vi "ActionVIOnCompile.vi"(8 "error in (no error)":errorcluster, 11 "Device Item Ref in":T1 format="%.0x") -> (0 "error out":errorcluster)   [LabVIEW 2020, in "PXI-2514 System Explorer.lvlib"]
uses:
  PXI-2514 System Explorer.lvlib
  <vilib>/NI VeriStand/Custom Device API/Custom Device Item Ref.ctl
  Shared/Compiled.Settings.ctl
  Shared/Constants.vi
  <vilib>/NI VeriStand/Custom Device API/Get Item Property (U16).vi
  <vilib>/NI VeriStand/Custom Device API/Get Item Property (String).vi
  <vilib>/NI VeriStand/Custom Device Tools/Custom Device Utility Library/NI VeriStand - Search for Item by Name.vi
  <vilib>/NI VeriStand/Custom Device API/Set Item Property (Variant).vi
  <vilib>/NI VeriStand/Custom Device Tools/Custom Device Utility Library/Custom Device Utility Library.lvlib
  <vilib>/NI VeriStand/Custom Device API/Custom Device API.lvlib
  <vilib>/NI/NIVS Inline Async API/_Data Access System Explorer/Data Access System Explorer.lvlib
  Shared/PXI-2514 Shared.lvlib
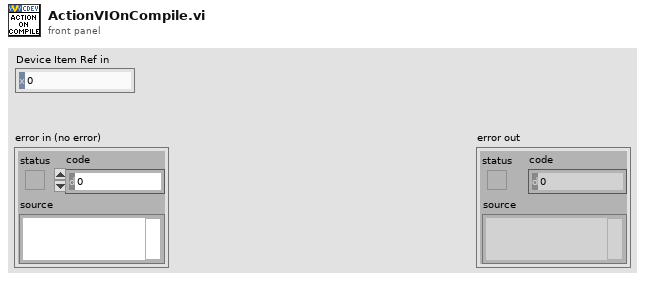
[diagram p1: front panel]
types:
  T1 = typedef "Custom Device API.lvlib/Custom Device Item Ref.ctl" = u64
  T2 = cluster{"Name":string, "Type":enum16{"Output/Write", "Input/Read", "Input/ReadWrite"}, "VS Refs":T1[]}
  T3 = enum16{"Output/Write", "Input/Read", "Input/ReadWrite"}
  T4 = typedef "PXI-2514 Shared.lvlib/Compiled.Settings.ctl" = cluster{"Name":string, "Async Init Timeout":u16, "Hardware Device Name":string}
  T5 = typedef "Custom Device API.lvlib/Custom Device Item Info.ctl" = cluster{"Name":string, "Is Channel":bool, "GUID":string, "Is Waveform":bool}
  T6 = cluster{"Name":string, "Type":enum16{"Output/Write", "Input/Read", "Input/ReadWrite"}, "VS Refs":T1[]}[]
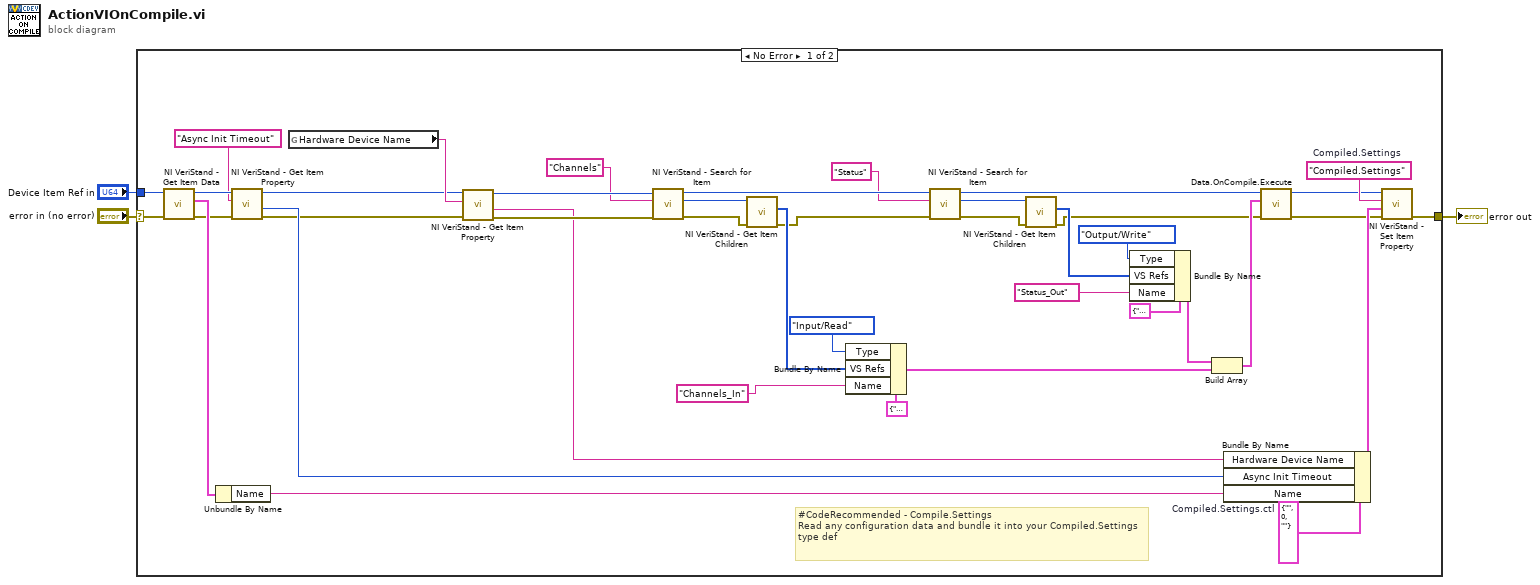
[diagram p0: block diagram]
diagram:
  n1 = case shown="No Error" "error in (no error)" {
    selector: "error in (no error)" -> [w37 w45]
    tunnel: [w38 w45] -> w2
    tunnel: "Device Item Ref in" -> [w36 _]
    frame No Error {
      w17 = T4 {"Name"="", "Async Init Timeout"=0, "Hardware Device Name"=""}  # Compiled.Settings.ctl
      w40 = "Compiled.Settings"  # Compiled.Settings
      # "#CodeRecommended - Compile.Settings\nRead any configuration data and bundle it into your Compiled.Settings type def"
      n2 = call <vilib>:"NI VeriStand - Get Item Data.vi"("error in (no error)"=w37, "Item Ref in"=w36) -> ("error out"=w16:errorcluster, "Item Info"=w35:T5, "Item Ref out"=w15:T1)  [unwired: 6 in, 1 out]
      n3 = Unbundle By Name(w35) -> ("Name"=w34:string)
      n4 = call-poly <vilib>:"NI VeriStand - Get Item Property.vi"("error in (no error)"=w16, "Property Name"="Async Init Timeout", "Item Ref in"=w15) -> ("error out"=w9:errorcluster, "Value"=w13:u16, "Item Ref out"=w11:T1)  [unwired: 5 in, 1 out]
      n5 = global read "Constants.vi" "Hardware Device Name"() -> (w12:string)
      n6 = call-poly <vilib>:"NI VeriStand - Get Item Property.vi"("error in (no error)"=w9, "Property Name"=w12, "Item Ref in"=w11) -> ("error out"=w8:errorcluster, "Value"=w7:string, "Item Ref out"=w10:T1)  [unwired: 5 in, 1 out]
      n7 = call-poly <vilib>:"NI VeriStand - Search for Item.vi"("error in"=w8, "Item Name"="Channels", "Section Ref in"=w10) -> ("error out"=w44:errorcluster, "Item Ref"=w43:T1, "Section Ref out"=w21:T1)  [unwired: 5 in, 1 out]
      n8 = call <vilib>:"NI VeriStand - Get Item Children.vi"("error in (no error)"=w44, "Item Ref in"=w43) -> ("error out"=w20:errorcluster, "Child Refs"=w33:T1[])  [unwired: 6 in, 2 out]
      n9 = Bundle By Name(cluster=T2 {"Name"="", "Type"=enum."Output/Write", "VS Refs"=[]} ("Group"), "Type"=T3."Input/Read", "VS Refs"=w33, "Name"="Channels_In" ("Item Name")) -> (w24:T2)
      n10 = call-poly <vilib>:"NI VeriStand - Search for Item.vi"("error in"=w20, "Item Name"="Status", "Section Ref in"=w21) -> ("error out"=w41:errorcluster, "Item Ref"=w42:T1, "Section Ref out"=w22:T1)  [unwired: 5 in, 1 out]
      n11 = call <vilib>:"NI VeriStand - Get Item Children.vi"("error in (no error)"=w41, "Item Ref in"=w42) -> ("error out"=w23:errorcluster, "Child Refs"=w28:T1[])  [unwired: 6 in, 2 out]
      n12 = Bundle By Name(cluster=T2 {"Name"="", "Type"=enum."Output/Write", "VS Refs"=[]} ("Group"), "Type"=T3."Output/Write", "VS Refs"=w28, "Name"="Status_Out" ("Item Name")) -> (w30:T2)
      n13 = Build Array(w30, w24) -> (w27:T6)
      n14 = Bundle By Name(cluster=w17, "Hardware Device Name"=w7, "Async Init Timeout"=w13, "Name"=w34) -> (w39:T4)
      n15 = call <vilib>:"Data.OnCompile.Execute.vi"("error in"=w23, "VS Ref Groups"=w27, "Custom Device Ref"=w22) -> ("error out"=w19:errorcluster, "Custom Device Ref"=w18:T1)  [unwired: 7 in]
      n16 = call-poly <vilib>:"NI VeriStand - Set Item Property.vi"("error in (no error)"=w19, "Value"=w39, "Property Name"=w40, "Item Ref in"=w18) -> ("error out"=w38:errorcluster)  [unwired: 5 in, 2 out]
    }
    frame Error {
    }
  }
  "error out" <- w2
